vi "Do.vi"(8 "error in (no error)":errorcluster, 10 "Actor in":refnum<class "Actor.lvclass">, 11 "JoinGame Msg":refnum<class "JoinGame Msg.lvclass">) -> (0 "error out":errorcluster, 2 "Actor out":refnum<class "Actor.lvclass">)   [LabVIEW 2014, in "GoBang.lvlib" / "JoinGame Msg.lvclass"]
doc: "This VI delivers the message to the actor by calling the appropriate method(s) on the actor."
uses:
  JoinGame Msg.lvclass
  Server/CS++GoBangServer.lvclass
  CSPP_Core/Actors/CS++PVMonitor Messages/CS++PVUpdate Msg/CS++PVUpdate Msg.lvclass
  CSPP_Core/Classes/CS++ProcessVariables/ProcessVariable/PV.lvclass
  <vilib>/ActorFramework/Actor/Actor.lvclass
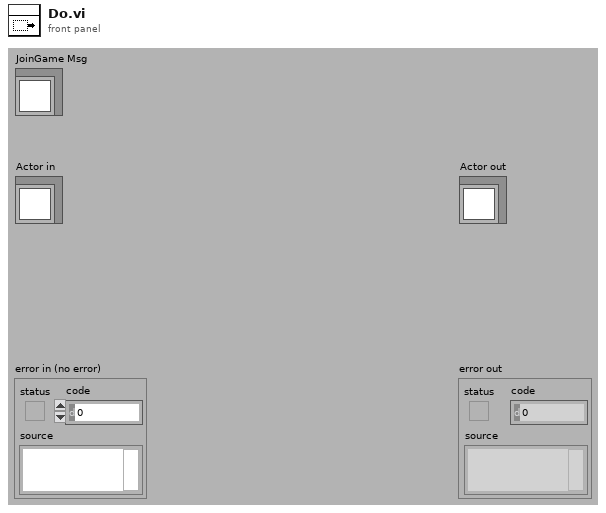
[diagram p1: front panel]
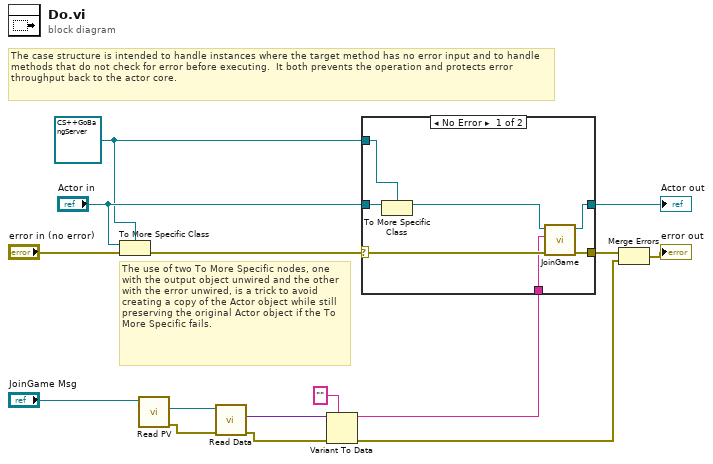
[diagram p0: block diagram]
diagram:
  w10 = refnum<class "CS++GoBangServer.lvclass"> refnum ("Actor in")
  # "The use of two To More Specific nodes, one with the output object unwired and the other with the error unwired, is a trick to avoid creating a copy of the Actor object while still preserving the original Actor object if the To More Specific fails."
  # "The case structure is intended to handle instances where the target method has no error input and to handle methods that do not check for error before executing.  It both prevents the operation and protects error throughput back to the actor core."
  n1 = To More Specific Class(target class=w10, reference="Actor in", error in="error in (no error)") -> (error out=w14:errorcluster)  [unwired: 1 out]
  n2 = call "Read PV.vi"("CS++PVUpdate Msg in"="JoinGame Msg") -> ("error out"=w4:errorcluster, "PV"=w8:refnum<class "PV.lvclass">)  [unwired: 8 in, 1 out]
  n3 = call "Read Data.vi"("error in (no error)"=w4, "PV in"=w8) -> ("error out"=w3:errorcluster, "Data"=w7:variant)  [unwired: 7 in, 1 out]
  n4 = Variant To Data(error in=w3, type="", Variant=w7) -> (data=w6:string, error out=w1:errorcluster)
  n5 = case shown="No Error" w14 {
    selector: w14 -> [w20 w24]
    tunnel: [w22 w24] -> w13
    tunnel: [w21 w23] -> w12
    tunnel: "Actor in" -> [w19 w23]
    tunnel: w10 -> [w18 _]
    tunnel: w6 -> [w16 _]
    frame No Error {
      n6 = To More Specific Class(target class=w18, reference=w19) -> (specific class reference=w17:refnum<class "CS++GoBangServer.lvclass">)  [unwired: 1 in, 1 out]
      n7 = call-dynamic "JoinGame.vi"("error in (no error)"=w20, "PlayerName"=w16, "CS++GoBangServer in"=w17) -> ("error out"=w22:errorcluster, "CS++GoBangServer out"=w21:refnum<class "CS++GoBangServer.lvclass">)  [unwired: 7 in]
    }
    frame Error {
      # "If type check fails, pass the original object out again."
    }
  }
  "Actor out" <- w12
  n8 = Merge Errors(w13, w1) -> (→"error out":errorcluster)
